vi "EX_Set_V_A.vi"(8 "错误输入（无错误）":errorcluster, 9 "current":string, 10 "voltage":string, 11 "VISA resource name":refnum<visa-resource-name> caption="VISA资源名称") -> (0 "error out":errorcluster caption="错误输出", 3 "VISA资源名称输出":refnum<visa-resource-name>)   [LabVIEW 2017]
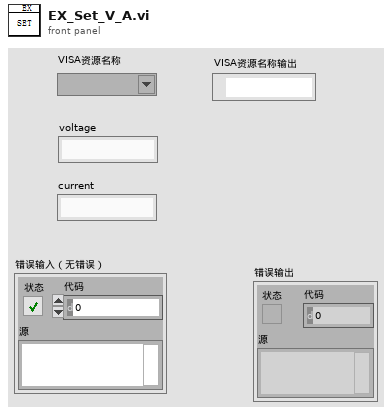
[diagram p1: front panel]
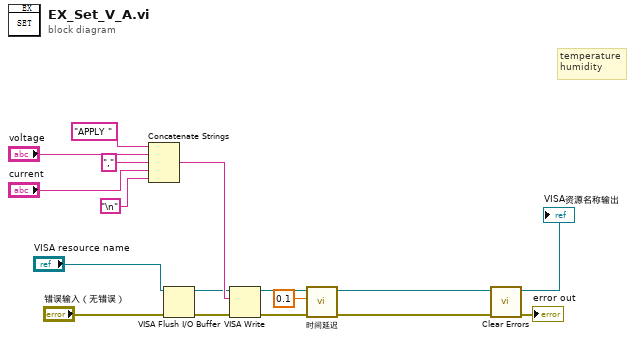
[diagram p0: block diagram]
diagram:
  # "temperature\nhumidity"
  n1 = Concatenate Strings("APPLY ", "voltage", "," ("字符串"), "current", "\n") -> (w12:string)
  n2 = VISA Flush I/O Buffer(VISA resource name="VISA resource name", error in (no error)="错误输入（无错误）") -> (VISA resource name out=w3:refnum<visa-resource-name>, error out=w2:errorcluster)  [unwired: 1 in]
  n3 = VISA Write(VISA resource name=w3, write buffer=w12, error in (no error)=w2) -> (VISA resource name out=→"VISA资源名称输出":refnum<visa-resource-name>, error out=w15:errorcluster)  [unwired: 1 out]
  n4 = call "时间延迟"("error in (no error)"=w15, "Delay Time (s)"=0.1) -> ("error out"=w6:errorcluster)  [unwired: 9 in]
  n5 = call <vilib>:"Clear Errors.vi"("error in (no error)"=w6) -> ("error out"=→"error out":errorcluster)  [unwired: 5 in, 1 out]
